vi "VendingMachine2.vi"() -> ()   [LabVIEW 2010]
panel:
  in  "dropCoinButton":bool
  in  "Kabooom":bool
  out "Result":string
  in  "spend1Coin":bool
  out "coinsDropped":i32
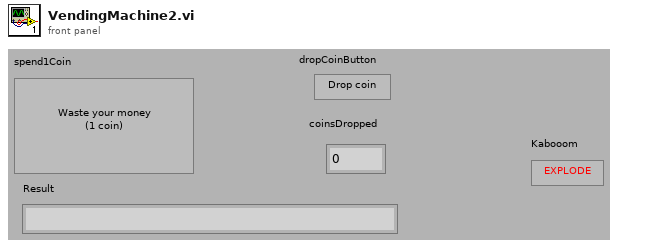
[diagram p1: front panel]
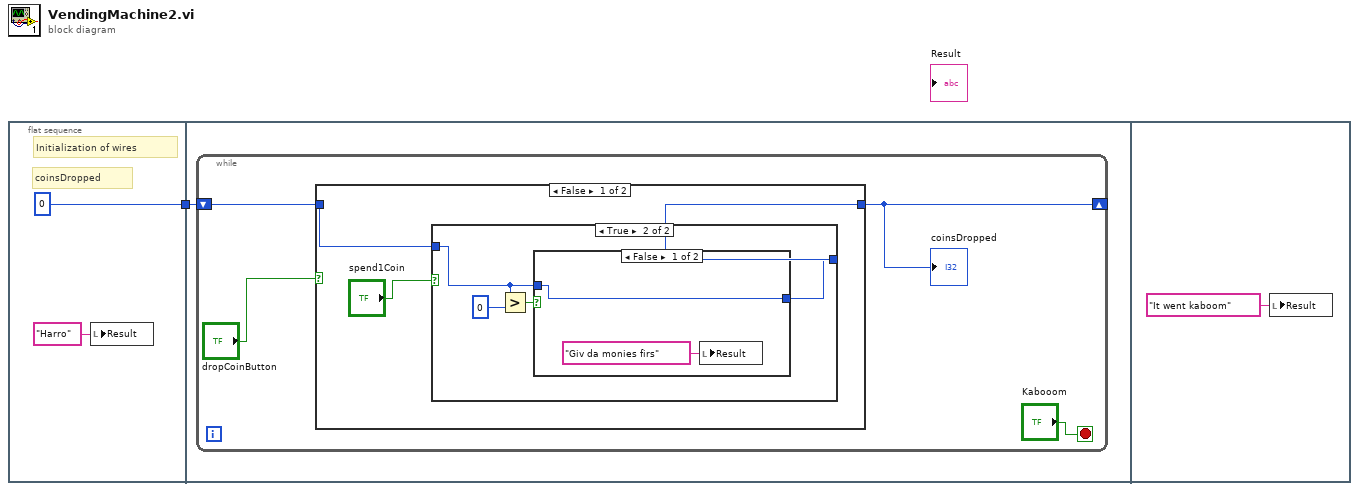
[diagram p0: block diagram]
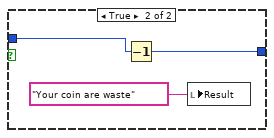
[diagram p3: hidden frame]
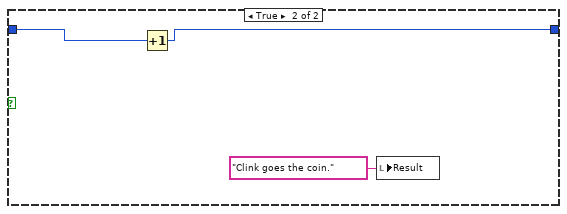
[diagram p4: hidden frame]
diagram:
  n1 = flat-sequence {
    tunnel: [0] -> w1
    tunnel: w1 -> [w4]
    frame #0 {
      # "Initialization of wires"
      # "coinsDropped"
      n2 = local write "Result"("Harro" ("Result")) -> ()
    }
    frame #1 {
      n3 = while {
        shift-right: [w5] -> _
        shift-left: w4 -> [w7]
        stop <- "Kabooom" stop-if-true
        n4 = case shown="False" "dropCoinButton" {
          tunnel: [w9 w23] -> w5
          tunnel: w7 -> [w11 w24]
          frame False {
            n5 = case shown="True" "spend1Coin" {
              tunnel: w11 -> [w12 w14]
              tunnel: [w12 w13] -> w9
              frame False {
              }
              frame True {
                n6 = Greater?(x=w14, y=0) -> (0:w15:bool)
                n7 = case shown="False" w15 {
                  tunnel: w14 -> [w18 w20]
                  tunnel: [w18 w19] -> w13
                  frame False {
                    n8 = local write "Result"("Giv da monies firs" ("Result")) -> ()
                  }
                  frame True {
                    n9 = Decrement(x=w20) -> (x-1=w19:i32)
                    n10 = local write "Result"("Your coin are waste" ("Result")) -> ()
                  }
                }
              }
            }
          }
          frame True {
            n11 = Increment(x=w24) -> (x+1=w23:i32)
            n12 = local write "Result"("Clink goes the coin." ("Result")) -> ()
          }
        }
        "coinsDropped" <- w5
      }
    }
    frame #2 {
      n13 = local write "Result"("It went kaboom" ("Result")) -> ()
    }
  }
